vi "RunWaves.vi"(6 "Analogue Out":waveform(dbl)[](array[waveform]), 7 "Digital Out":digitalwaveform[](array[waveform]), 9 "Microscope Settings":T1={"Mode"=enum."X", "Slit"={"Scanning Mode"=0.0, "Slit Width /%"=0.0}, "Colour"=[], "Exposure/ms"=0.0, "Piezo Position /um"=0.0, "ROI"={"X"={"Start /px"=0.0, "Step /px"=0.0, "Range /px"=0.0}, "Y"={"Start /px"=0.0, "Step /px"=0.0, "Range /px"=0.0}, "Z "={"Start /um"=0.0, "Step/um"=0.0, "Range /um"=0.0}, "T "={"Start /s"=0.0, "Step /s"=0.0, "Range /s"=0.0}}, "Samples per millisecond"=0.0, "Relax/ms"=0.0, "Readout Direction"=0.0, "Trigger Source"=0.0, "Camera Delay /ms"=0.0, "Under Scan /ms"=0.0, "Calibration Coordinates"={"Top Left"=[], "Top Right"=[], "Bottom Left"=[], "Bottom Right"=[], "Waveforms"={"Analogue Out"=[], "Digital Out"=[]}}} {"Under Scan /ms" min=0.0 max=10.0 step=0.05; "ROI"."T"."Range /s" min=0.0 max=10.0 step=0.05; "ROI"."T"."Step /s" min=0.0 max=10.0 step=0.05; "ROI"."T"."Start /s" min=0.0 max=10.0 step=0.05; "ROI"."X"."Range /px" min=0.0 max=10.0 step=0.05; "ROI"."X"."Step /px" min=0.0 max=10.0 step=0.05; "ROI"."X"."Start /px" min=0.0 max=10.0 step=0.05; "ROI"."Y"."Range /px" min=0.0 max=10.0 step=0.05; "ROI"."Y"."Step /px" min=0.0 max=10.0 step=0.05; "ROI"."Y"."Start /px" min=0.0 max=10.0 step=0.05; "ROI"."Z"."Range /um" min=0.0 max=10.0 step=0.05; "ROI"."Z"."Step/um" min=0.0 max=10.0 step=0.05; "ROI"."Z"."Start /um" min=0.0 max=10.0 step=0.05; "Colour"."Filter" items=["Empty"=1, ""=2, ""=3, "561"=4, ""=5, "488"=6]; "Camera Delay /ms" min=0.0 max=10.0 step=0.05; "Trigger Source" items=["Internal"=1.0, "External"=2.0]; "Readout Direction" items=["Forward"=1.0, "Backward"=2.0]; "Slit"."Scanning Mode" items=["Full Frame"=1.0, "Slit Scanning"=12.0]; "Piezo Position /um" min=0.0 max=10.0 step=0.05}, 10 "Digital In":refnum<k21>, 11 "Analogue  in":refnum<k21>) -> (2 "Digital Out":refnum<k21>, 3 "Analogue Out":refnum<k21>)   [LabVIEW 2016]
uses:
  controls/Microscope Settings.ctl
  <vilib>/DAQmx/write.llb/DAQmx Write (Digital 1D Wfm NChan NSamp).vi
  <vilib>/DAQmx/write.llb/DAQmx Write (Analog 1D Wfm NChan NSamp).vi
  <vilib>/Waveform/WDTOps.llb/WDT Number of Waveform Samples DBL.vi
  <vilib>/DAQmx/configure/timing.llb/DAQmx Timing (Sample Clock).vi
  <vilib>/Waveform/DWDTOps.llb/DWDT Uncompress Digital.vi
  <vilib>/DAQmx/miscellaneous.llb/DAQmx Fill In Error Info.vi
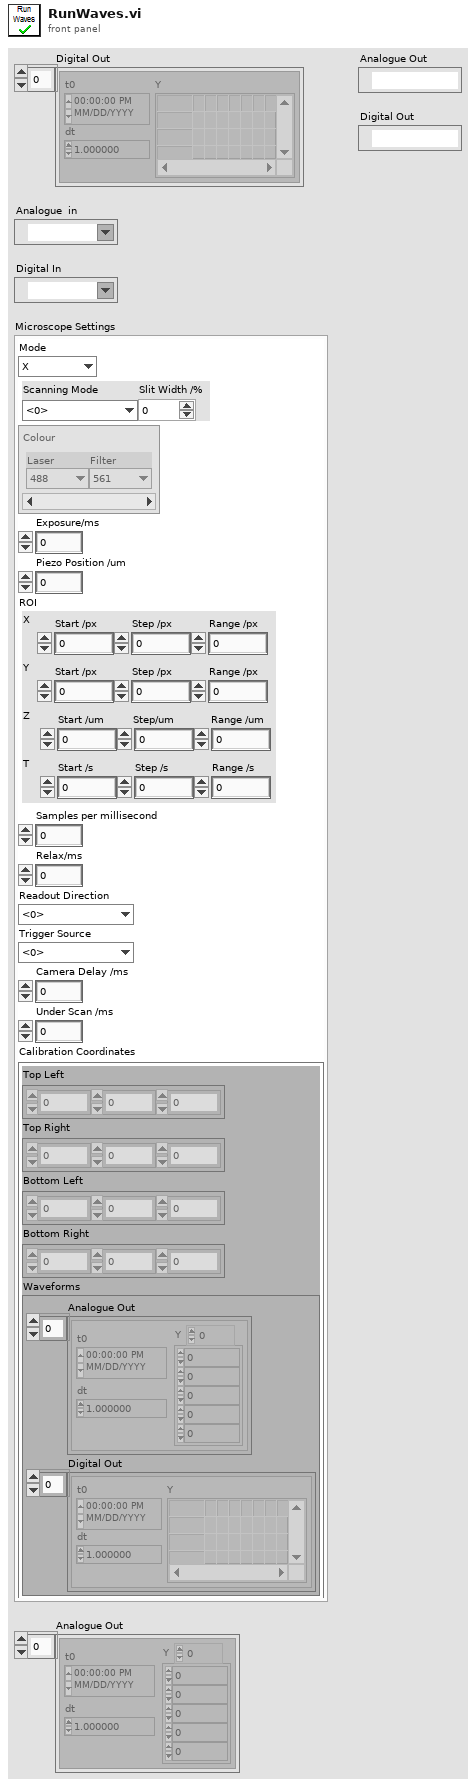
[diagram p1: front panel]
types:
  T1 = typedef "Microscope Settings.ctl" = cluster{"Mode":enum16{"Brightfield", "X", "XY", "XYZ", "XYZT", "XYZC", "Tweezers", "Virus"}, "Slit":cluster{"Scanning Mode":dbl, "Slit Width /%":dbl}, "Colour":cluster{"Laser":enum16{"Brightfield", "445", "488", "561", "647"}, "Filter":u16}[], "Exposure/ms":dbl, "Piezo Position /um":dbl, "ROI":cluster{"X":cluster{"Start /px":dbl, "Step /px":dbl, "Range /px":dbl}, "Y":cluster{"Start /px":dbl, "Step /px":dbl, "Range /px":dbl}, "Z ":cluster{"Start /um":dbl, "Step/um":dbl, "Range /um":dbl}, "T ":cluster{"Start /s":dbl, "Step /s":dbl, "Range /s":dbl}}, "Samples per millisecond":dbl, "Relax/ms":dbl, "Readout Direction":dbl, "Trigger Source":dbl, "Camera Delay /ms":dbl, "Under Scan /ms":dbl, "Calibration Coordinates":cluster{"Top Left":dbl[], "Top Right":dbl[], "Bottom Left":dbl[], "Bottom Right":dbl[], "Waveforms":cluster{"Analogue Out":waveform(dbl)[], "Digital Out":digitalwaveform[]}}}
  T2 = enum16{"Brightfield", "X", "XY", "XYZ", "XYZT", "XYZC", "Tweezers", "Virus"}
  T3 = cluster{"Start /s":dbl, "Step /s":dbl, "Range /s":dbl}
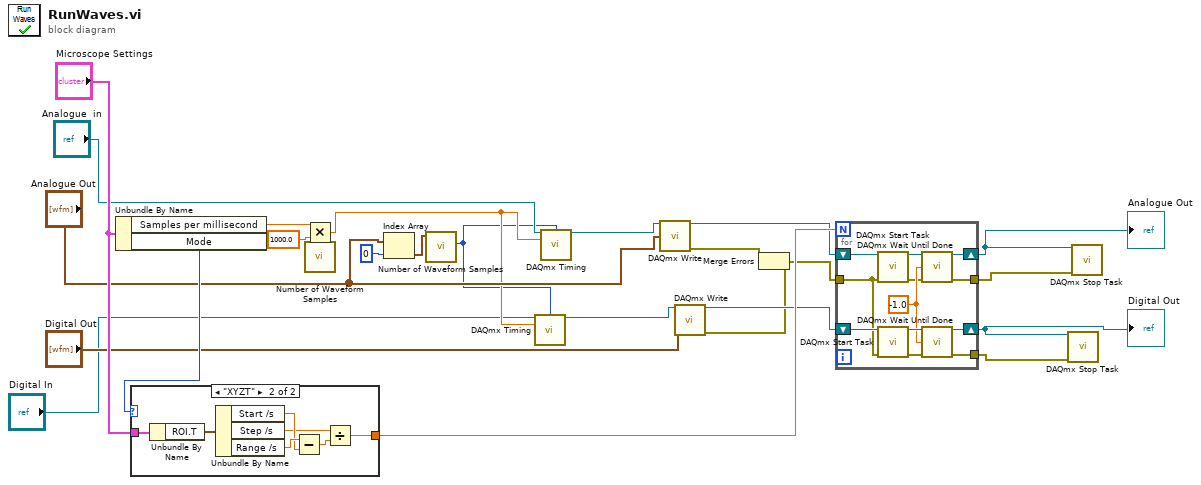
[diagram p0: block diagram]
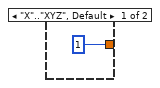
[diagram p2: hidden frame]
diagram:
  n1 = Unbundle By Name("Microscope Settings") -> ("Samples per millisecond"=w2:dbl, "Mode"=w19:T2)
  n2 = case shown="\"XYZT\"" w19 {
    tunnel: [1 w26] -> w20
    tunnel: "Microscope Settings" -> [_ w32]
    frame "X".."XYZ", Default {
    }
    frame "XYZT" {
      n3 = Unbundle By Name(w32) -> ("ROI.T"=w31:T3)
      n4 = Unbundle By Name(w31) -> ("Start /s"=w29:dbl, "Step /s"=w27:dbl, "Range /s"=w30:dbl)
      n5 = Subtract(x=w30, y=w29) -> (x-y=w28:dbl)
      n6 = Divide(x=w27, y=w28) -> (x/y=w26:dbl)
    }
  }
  n7 = Multiply(x=w2, y=1000.0) -> (x*y=w8:dbl)
  n8 = call-poly <vilib>:"Number of Waveform Samples.vi"() -> ()  [unwired: 9 in, 3 out]
  n9 = Index Array(array="Analogue Out", index=0) -> (element=w4:waveform(dbl))
  n10 = call-poly <vilib>:"Number of Waveform Samples.vi"("waveform in"=w4) -> ("number of samples"=w5:i32)  [unwired: 8 in, 2 out]
  n11 = call-poly <vilib>:"DAQmx Timing.vi"("task/channels in"="Digital In", "samples per channel"=w5, "rate"=w8) -> ("task out"=w10:refnum<k21>)  [unwired: 11 in, 1 out]
  n12 = call-poly <vilib>:"DAQmx Timing.vi"("task/channels in"="Analogue  in", "samples per channel"=w5, "rate"=w8) -> ("task out"=w9:refnum<k21>)  [unwired: 11 in, 1 out]
  n13 = call-poly <vilib>:"DAQmx Write.vi"("task/channels in"=w9, "data"="Analogue Out") -> ("task out"=w13:refnum<k21>, "error out"=w11:errorcluster)  [unwired: 11 in, 1 out]
  n14 = call-poly <vilib>:"DAQmx Write.vi"("task/channels in"=w10, "data"="Digital Out") -> ("task out"=w14:refnum<k21>, "error out"=w12:errorcluster)  [unwired: 11 in, 1 out]
  n15 = Merge Errors(w11, w12) -> (w15:errorcluster)
  n16 = for {
    N: w20 -> [_]
    tunnel: w15 -> [w38]
    shift-right: [w41] -> w21
    shift-left: w13 -> [w44]
    shift-right: [w39] -> w24
    shift-left: w14 -> [w43]
    tunnel: [w34] -> w23
    tunnel: [w33] -> w22
    w37 = -1.0 ("timeout (sec)")
    n17 = call <vilib>:"DAQmx Start Task.vi"("task/channels in"=w44, "error in"=w38) -> ("task out"=w42:refnum<k21>, "error out"=w36:errorcluster)  [unwired: 12 in]
    n18 = call <vilib>:"DAQmx Start Task.vi"("task/channels in"=w43, "error in"=w38) -> ("task out"=w40:refnum<k21>, "error out"=w35:errorcluster)  [unwired: 12 in]
    n19 = call <vilib>:"DAQmx Wait Until Done.vi"("task/channels in"=w42, "timeout (sec)"=w37, "error in"=w36) -> ("task out"=w41:refnum<k21>, "error out"=w33:errorcluster)  [unwired: 11 in]
    n20 = call <vilib>:"DAQmx Wait Until Done.vi"("task/channels in"=w40, "timeout (sec)"=w37, "error in"=w35) -> ("task out"=w39:refnum<k21>, "error out"=w34:errorcluster)  [unwired: 11 in]
  }
  "Digital Out" <- w24
  "Analogue Out" <- w21
  n21 = call <vilib>:"DAQmx Stop Task.vi"("task/channels in"=w24, "error in"=w23) -> ()  [unwired: 12 in, 2 out]
  n22 = call <vilib>:"DAQmx Stop Task.vi"("task/channels in"=w21, "error in"=w22) -> ()  [unwired: 12 in, 2 out]
